vi "DriveModuleControl_TravTunePID_Dash.vi"(0 "Network Table Prefix":i32) -> (2 "TestDone":bool, 3 "TestInProcess":bool, 4 "Kp":dbl, 6 "Ki":dbl, 8 "Kd":dbl, 10 "PvStdDev":dbl, 12 "ConstDone":bool, 13 "Error":bool, 14 "PlantDone":bool, 15 "CoStdDev":dbl)   [LabVIEW 2023]
uses:
  <vilib>/Rock Robotics/Network Tables/NT Read Boolean.vi
  <vilib>/Rock Robotics/Network Tables/NT Read Number.vi
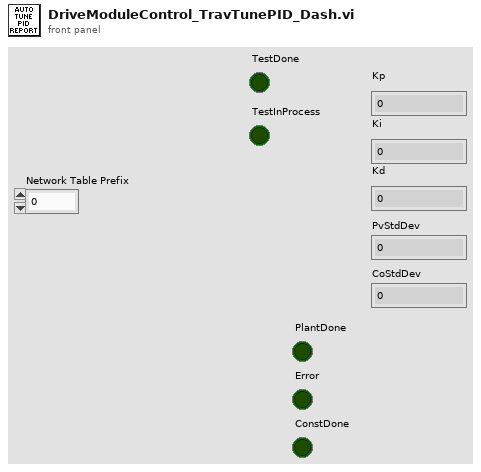
[diagram p1: front panel]
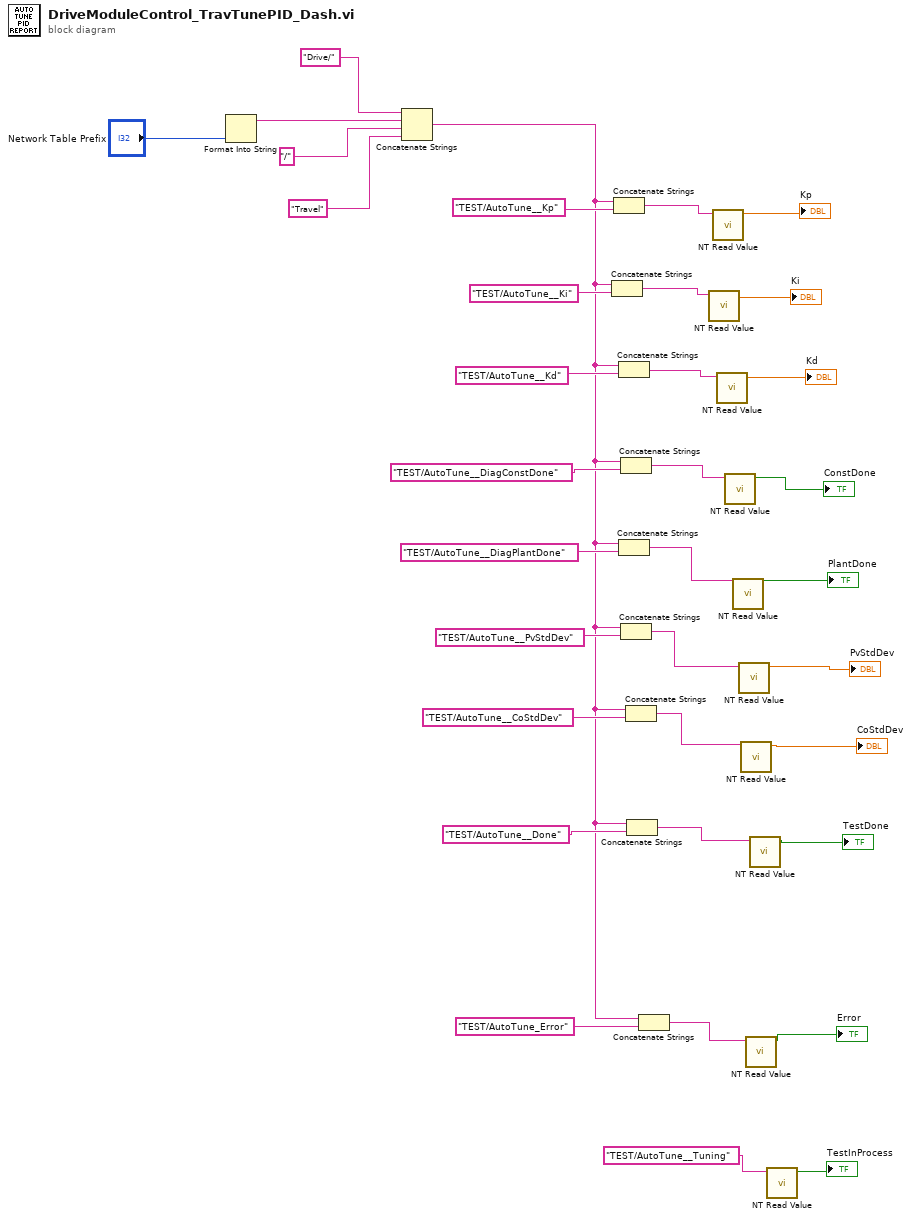
[diagram p0: block diagram]
diagram:
  n1 = Format Into String("Network Table Prefix") -> (resulting string=w4:string)  [unwired: 3 in, 1 out]
  n2 = Concatenate Strings("Drive/" ("string"), w4, "/" ("string"), "Travel" ("refnum name")) -> (w1:string)
  n3 = Concatenate Strings(w1, "TEST/AutoTune__Ki" ("name")) -> (w25:string)
  n4 = Concatenate Strings(w1, "TEST/AutoTune__Kp" ("name")) -> (w24:string)
  n5 = Concatenate Strings(w1, "TEST/AutoTune__Kd" ("name")) -> (w26:string)
  n6 = Concatenate Strings(w1, "TEST/AutoTune__DiagPlantDone" ("name")) -> (w32:string)
  n7 = Concatenate Strings(w1, "TEST/AutoTune__DiagConstDone" ("name")) -> (w28:string)
  n8 = Concatenate Strings(w1, "TEST/AutoTune__PvStdDev" ("name")) -> (w33:string)
  n9 = Concatenate Strings(w1, "TEST/AutoTune__CoStdDev" ("name")) -> (w34:string)
  n10 = Concatenate Strings(w1, "TEST/AutoTune__Done" ("name")) -> (w18:string)
  n11 = Concatenate Strings(w1, "TEST/AutoTune_Error" ("name")) -> (w17:string)
  n12 = call-poly <vilib>:"NT Read Value.vi"("name"=w25) -> ("value"=→"Ki":dbl)  [unwired: 8 in, 2 out]
  n13 = call-poly <vilib>:"NT Read Value.vi"("name"=w24) -> ("value"=→"Kp":dbl)  [unwired: 8 in, 2 out]
  n14 = call-poly <vilib>:"NT Read Value.vi"("name"=w26) -> ("value"=→"Kd":dbl)  [unwired: 8 in, 2 out]
  n15 = call-poly <vilib>:"NT Read Value.vi"("name"=w28) -> ("value"=→"ConstDone":bool)  [unwired: 8 in, 2 out]
  n16 = call-poly <vilib>:"NT Read Value.vi"("name"=w32) -> ("value"=→"PlantDone":bool)  [unwired: 8 in, 2 out]
  n17 = call-poly <vilib>:"NT Read Value.vi"("name"=w33) -> ("value"=→"PvStdDev":dbl)  [unwired: 8 in, 2 out]
  n18 = call-poly <vilib>:"NT Read Value.vi"("name"=w34) -> ("value"=→"CoStdDev":dbl)  [unwired: 8 in, 2 out]
  n19 = call-poly <vilib>:"NT Read Value.vi"("name"=w17) -> ("value"=→"Error":bool)  [unwired: 8 in, 2 out]
  n20 = call-poly <vilib>:"NT Read Value.vi"("name"=w18) -> ("value"=→"TestDone":bool)  [unwired: 8 in, 2 out]
  n21 = call-poly <vilib>:"NT Read Value.vi"("name"="TEST/AutoTune__Tuning") -> ("value"=→"TestInProcess":bool)  [unwired: 8 in, 2 out]
